vi "AlliGator Select Decay Fit Parameter Scatterplot Type.vi"(8 "Error In":errorcluster) -> (0 "Error Out":errorcluster, 1 "Fit Parameter 2":T1=enum."tau_1", 2 "Fit Parameter 1":T1=enum."tau_1", 3 "Cancelled?":bool)   [LabVIEW 2021, in "AlliGator Decay Fit Parameter Map.lvlib"]
doc: "Dialog to select parameter 1 and parameter 2 to be computed for a Phasor Plot of the Phasor Graph."
uses:
  AlliGator Decay Fit Parameter Map.lvlib
  Fits/IRF(X)PSED/Decay Fit Parameters & Derived Quantities List v2.ctl
  Fits/Fits.lvlib
panel:
  in  "Cancel":bool
  in  "OK":bool
  in  "Fit Parameter 2":T1=enum."tau_2"
  in  "Fit Parameter 1":T1=enum."tau_1"
  # "Select parameters to export as scatter plot:\n\n- horizontal axis: Parameter 1\n- vertical axis: Parameter 2"
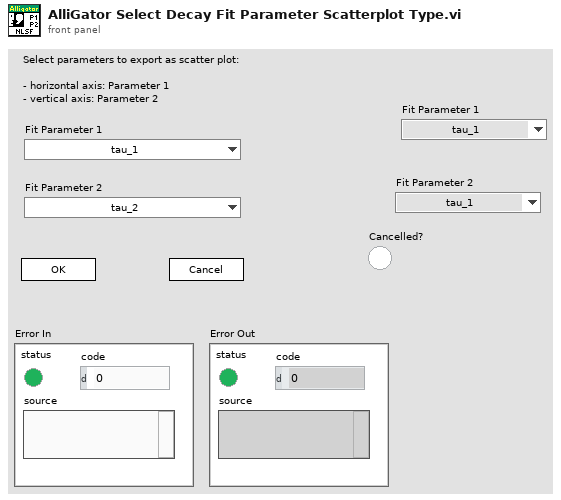
[diagram p1: front panel]
types:
  T1 = typedef "Fits.lvlib/Decay Fit Parameters & Derived Quantities List v2.ctl" = enum16{"Offset", "Baseline", "A_1", "tau_1", "A_2", "tau_2", "<tau>_a", "f1_a", "f2_a", "<tau>_i", "f1_i", "f2_i", "-", "R^2", "Chi^2"}
  T2 = enum32{"Invalid", "Standard", "Closed", "Hidden", "Minimized", "Maximized"}
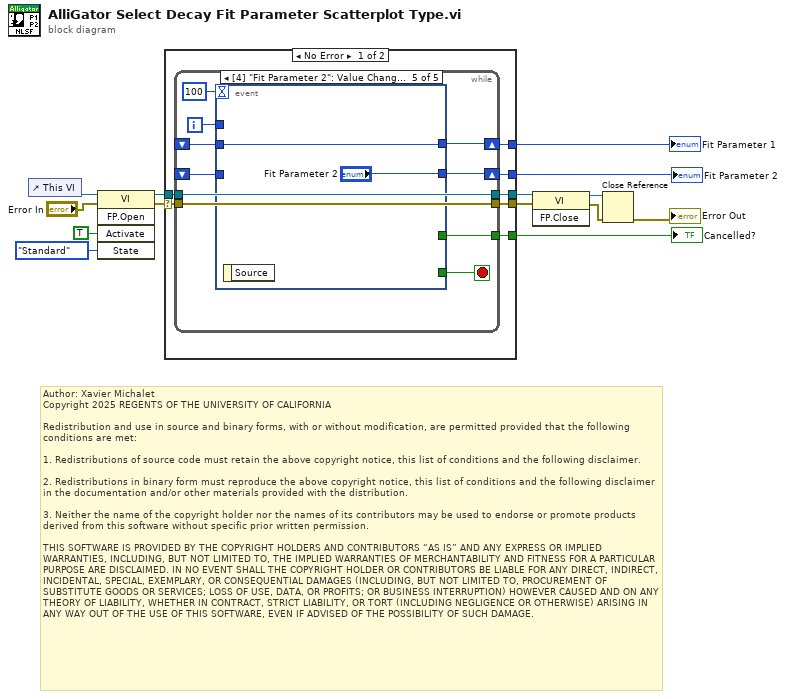
[diagram p0: block diagram]
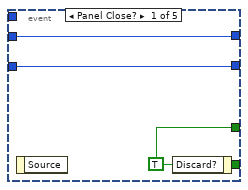
[diagram p2: hidden frame]
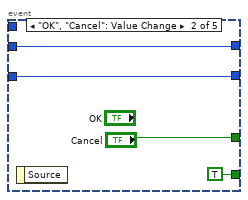
[diagram p3: hidden frame]
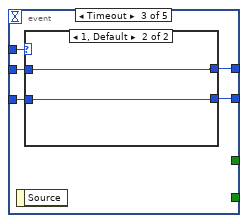
[diagram p4: hidden frame]
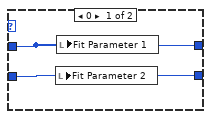
[diagram p5: hidden frame]
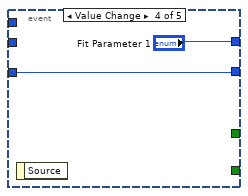
[diagram p6: hidden frame]
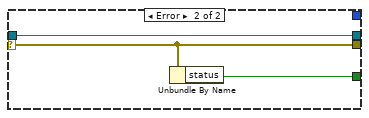
[diagram p7: hidden frame]
diagram:
  # "Author: Xavier Michalet\nCopyright 2025 REGENTS OF THE UNIVERSITY OF CALIFORNIA\n\nRedistribution and use in source and binary forms, with or without modification, are permitted provided that the following conditions are met:\n\n1. Redistributions of source code must retain the above copyright notice, this list of conditions and the following disclaimer.\n\n2. Redistributions in binary form must reproduce the above copyright notice, this list of conditions and the following disclaimer in the documentation and/or other materials provided with the distribution.\n\n3. Neither the name of the copyright holder nor the names of its contributors may be used to endorse or promote products derived from this software without specific prior written permission.\n\nTHIS SOFTWARE IS PROVIDED BY THE COPYRIGHT HOLDERS AND CONTRIBUTORS “AS IS” AND ANY EXPRESS OR IMPLIED WARRANTIES, INCLUDING, BUT NOT LIMITED TO, THE IMPLIED WARRANTIES OF MERCHANTABILITY AND FITNESS FOR A PARTICULAR PURPOSE ARE DISCLAIMED. IN NO EVENT SHALL THE COPYRIGHT HOLDER OR CONTRIBUTORS BE LIABLE FOR ANY DIRECT, INDIRECT, INCIDENTAL, SPECIAL, EXEMPLARY, OR CONSEQUENTIAL DAMAGES (INCLUDING, BUT NOT LIMITED TO, PROCUREMENT OF SUBSTITUTE GOODS OR SERVICES; LOSS OF USE, DATA, OR PROFITS; OR BUSINESS INTERRUPTION) HOWEVER CAUSED AND ON ANY THEORY OF LIABILITY, WHETHER IN CONTRACT, STRICT LIABILITY, OR TORT (INCLUDING NEGLIGENCE OR OTHERWISE) ARISING IN ANY WAY OUT OF THE USE OF THIS SOFTWARE, EVEN IF ADVISED OF THE POSSIBILITY OF SUCH DAMAGE."
  n1 = control-ref of="This VI"() -> (w9:refnum<vi>)
  n2 = invoke class="VI" method="FP.Open"(reference=w9, error in="Error In", "Activate"=TRUE ("Activate?"), "State"=T2."Standard") -> (reference out=w5:refnum<vi>, error out=w6:errorcluster)  [unwired: 1 in, 3 out]
  n3 = case shown="No Error" w6 {
    selector: w6 -> [w18 w53]
    tunnel: [w21 w52] -> w14
    tunnel: [w20 _] -> w13
    tunnel: [w19 _] -> w12
    tunnel: w5 -> [w17 w54]
    tunnel: [w16 w54] -> w4
    tunnel: [w15 w53] -> w3
    frame No Error {
      n4 = while {
        tunnel: [w30] -> w21
        shift-right: [w26] -> w20
        shift-left: _ -> [w27]
        shift-right: [w24] -> w19
        shift-left: _ -> [w25]
        tunnel: w18 -> [w22]
        tunnel: [w23] -> w16
        tunnel: w17 -> [w23]
        tunnel: [w22] -> w15
        i -> [w28]
        stop <- w31 stop-if-true
        n5 = event shown="[4] \"Fit Parameter 2\": Value Change" {
          selector: _ -> [_ _ _ _ _]
          dyn-events: _ -> [_ _ _ _ _]
          timeout: 100 -> [_ _ _ _ _]
          tunnel: [w34 TRUE ("Discard?") _ _ _] -> w31
          tunnel: [w34 "Cancel" _ _ _] -> w30
          tunnel: w28 -> [_ _ w43 _ _]
          tunnel: w27 -> [w33 w36 w42 _ w50]
          tunnel: [w33 w36 w41 "Fit Parameter 1" w50] -> w26
          tunnel: w25 -> [w32 w35 w40 w48 _]
          tunnel: [w32 w35 w39 w48 "Fit Parameter 2"] -> w24
          event Panel Close? {
            w34 = TRUE ("Discard?")
            n6 = event-data() -> ()  [unwired: 1 in, 1 out]
            n7 = event-data("Discard?"=w34) -> ()  [unwired: 1 in, 1 out]
          }
          event "OK", "Cancel": Value Change {
            n8 = event-data() -> ()  [unwired: 1 in, 1 out]
          }
          event Timeout {
            n9 = event-data() -> ()  [unwired: 1 in, 1 out]
            n10 = case shown="1, Default" w43 {
              tunnel: w42 -> [w45 w47]
              tunnel: [w45 w47] -> w41
              tunnel: w40 -> [w44 w46]
              tunnel: [w44 w46] -> w39
              frame 0 {
                n11 = local write "Fit Parameter 2"(w44) -> ()
                n12 = local write "Fit Parameter 1"(w45) -> ()
              }
              frame 1, Default {
              }
            }
          }
          event Value Change {
            n13 = event-data() -> ()  [unwired: 1 in, 1 out]
          }
          event Value Change {
            n14 = event-data() -> ()  [unwired: 1 in, 1 out]
          }
        }
      }
    }
    frame Error {
      n15 = Unbundle By Name(w53) -> ("status"=w52:bool)
    }
  }
  "Fit Parameter 1" <- w13
  "Fit Parameter 2" <- w12
  "Cancelled?" <- w14
  n16 = invoke class="VI" method="FP.Close"(reference=w4, error in=w3) -> (reference out=w2:refnum<vi>, error out=w1:errorcluster)  [unwired: 1 in, 1 out]
  n17 = Close Reference(reference=w2, error in (no error)=w1) -> (error out=→"Error Out":errorcluster)
